vi "配置网络.vi"() -> (0 "下载":bool, 2 "端口号":u16, 3 "IP":string)   [LabVIEW 2018]
panel:
  in  "Port":string="9000"
  in  "IP":string="192.168.1.2"
  in  "取消":bool
  in  "确认":bool
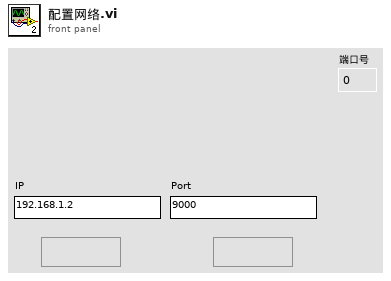
[diagram p1: front panel]
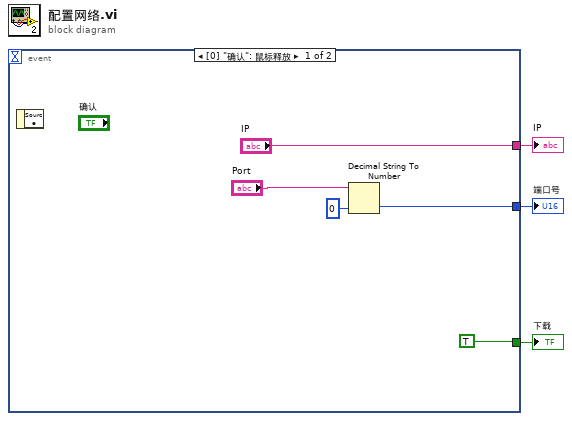
[diagram p0: block diagram]
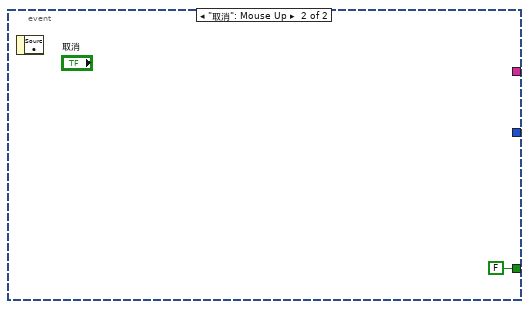
[diagram p2: hidden frame]
diagram:
  n1 = event shown="[0] \"确认\": 鼠标释放" {
    selector: _ -> [_ _]
    dyn-events: _ -> [_ _]
    timeout: _ -> [_ _]
    tunnel: ["IP" _] -> w3
    tunnel: [w5 _] -> w2
    tunnel: [TRUE FALSE] -> w1
    event "确认": Mouse Up {
      n2 = event-data() -> ()  [unwired: 1 in, 1 out]
      n3 = Decimal String To Number(string="Port", default (0L)=u16 0 ("默认(0 I32)")) -> (number=w5:u16)  [unwired: 1 in, 1 out]
    }
    event "取消": Mouse Up {
      n4 = event-data() -> ()  [unwired: 1 in, 1 out]
    }
  }
  "IP" <- w3
  "端口号" <- w2
  "下载" <- w1
